vi "Condition.vi"(8 "error in (no error)":errorcluster, 11 "IV_meas in":refnum<class "IV_meas.lvclass">) -> (0 "error out":errorcluster, 2 "Finish?":bool, 3 "IV_meas out":refnum<class "IV_meas.lvclass">)   [LabVIEW 2014, in "IV_meas.lvclass"]
uses:
  IV_meas.lvclass
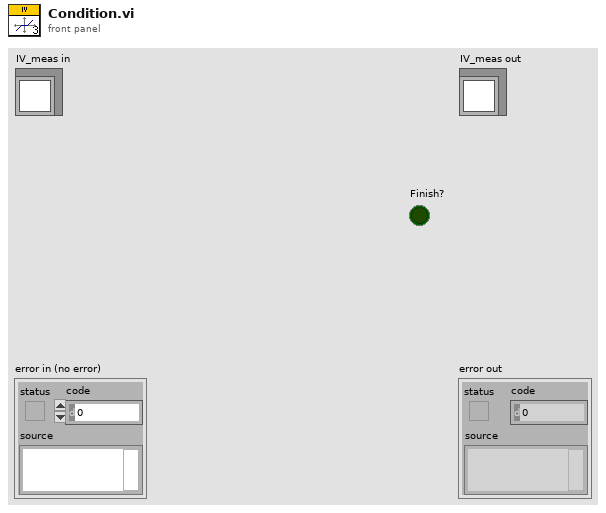
[diagram p1: front panel]
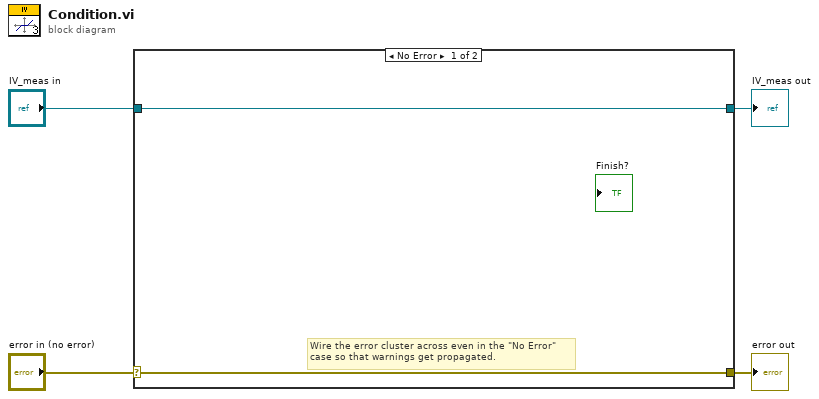
[diagram p0: block diagram]
diagram:
  n1 = case shown="No Error" "error in (no error)" {
    selector: "error in (no error)" -> [w5 w8]
    tunnel: [w5 w8] -> w3
    tunnel: [w6 w7] -> w1
    tunnel: "IV_meas in" -> [w6 w7]
    frame No Error {
      # "Wire the error cluster across even in the \"No Error\"\ncase so that warnings get propagated."
    }
    frame Error {
    }
  }
  "error out" <- w3
  "IV_meas out" <- w1
